vi "get_map_size.vi"(8 "error in (no error)":errorcluster, 10 "appended path":path, 11 "IntensityGraph in":refnum<vi>) -> (0 "error out":errorcluster, 2 "map size":cluster{dbl, dbl, dbl, dbl})   [LabVIEW 2012]
uses:
  <vilib>/Analysis/6fits.llb/Curve Fitting Criteria.ctl
  <vilib>/Utility/file.llb/Read From Spreadsheet File (string).vi
  <vilib>/Analysis/baseanly.llb/Mean (DBL).vi
  <vilib>/regexp/Match Regular Expression.xnode
  <vilib>/Analysis/NI_AALBase.lvlib
  <vilib>/Analysis/NI_AALPro.lvlib
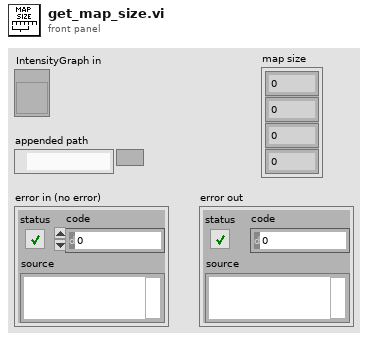
[diagram p1: front panel]
types:
  T1 = typedef "NI_AALPro.lvlib/Curve Fitting Criteria.ctl" = u16
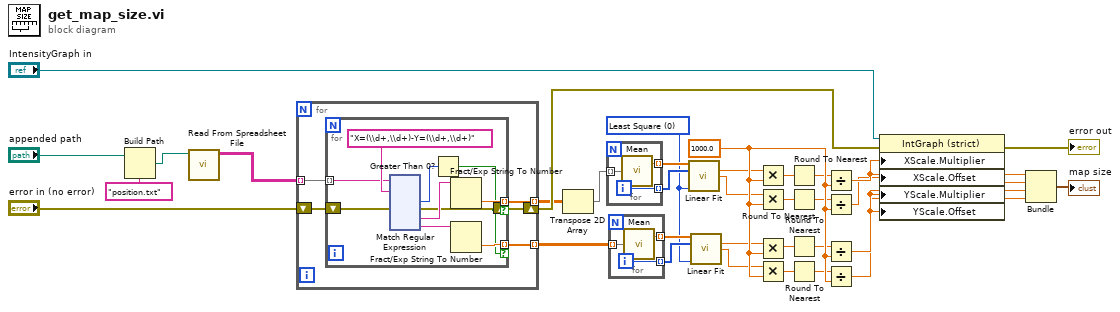
[diagram p0: block diagram]
diagram:
  w32 = 1000.0 ("y")
  w6 = T1 0 items=["Least Square", "Least Absolute Residual", "Bisquare"] ("method")
  n1 = Build Path(base path="appended path", name or relative path="position.txt") -> (appended path=w8:path)
  n2 = call-poly <vilib>:"Read From Spreadsheet File.vi"("file path (dialog if empty)"=w8) -> ("all rows"=w10:string[][])  [unwired: 6 in, 4 out]
  n3 = for {
    tunnel: w10 -> [w39] mode=indexing
    tunnel: [w38] -> w15 mode=indexing
    tunnel: [w37] -> w13 mode=indexing
    shift-right: [w36] -> w27
    shift-left: "error in (no error)" -> [w35]
    n4 = for {
      tunnel: w39 -> [w48] mode=indexing
      tunnel: [w46] -> w38 mode=indexing if=w42
      tunnel: [w45] -> w37 mode=indexing if=w42
      shift-right: [w41] -> w36
      shift-left: w35 -> [w40]
      n5 = xnode "Match Regular Expression"("input string"=w48, "regular expression"="X=(\\d+,\\d+)-Y=(\\d+,\\d+)", "error in"=w40) -> ("offset past match"=w43:i32, "error out"=w41:errorcluster, "submatch 1"=w44:string, "submatch 2"=w47:string)  [unwired: 3 in, 3 out]
      n6 = Greater Than 0?(x=w43) -> (x > 0?=w42:bool)
      n7 = Fract/Exp String To Number(string=w44) -> (number=w46:dbl)  [unwired: 3 in, 1 out]
      n8 = Fract/Exp String To Number(string=w47) -> (number=w45:dbl)  [unwired: 3 in, 1 out]
    }
  }
  n9 = Transpose 2D Array(2D array=w15) -> (transposed array=w14:dbl[][])
  n10 = for {
    tunnel: w14 -> [w166] mode=indexing
    tunnel: [w165] -> w17 mode=indexing
    tunnel: [w164] -> w11 mode=indexing
    i -> [w164]
    n11 = call-poly <vilib>:"Mean.vi"("X"=w166) -> ("mean"=w165:dbl)  [unwired: 1 out]
  }
  n12 = for {
    tunnel: w13 -> [w169] mode=indexing
    tunnel: [w168] -> w16 mode=indexing
    tunnel: [w167] -> w12 mode=indexing
    i -> [w167]
    n13 = call-poly <vilib>:"Mean.vi"("X"=w169) -> ("mean"=w168:dbl)  [unwired: 1 out]
  }
  n14 = call <vilib>:"Linear Fit.vi"("Y"=w17, "X"=w11, "method"=w6) -> ("slope"=w18:dbl, "intercept"=w19:dbl)  [unwired: 8 in, 3 out]
  n15 = call <vilib>:"Linear Fit.vi"("Y"=w16, "X"=w12, "method"=w6) -> ("slope"=w20:dbl, "intercept"=w21:dbl)  [unwired: 8 in, 3 out]
  n16 = Multiply(x=w18, y=w32) -> (x*y=w22:dbl)
  n17 = Multiply(x=w19, y=w32) -> (x*y=w23:dbl)
  n18 = Multiply(x=w20, y=w32) -> (x*y=w25:dbl)
  n19 = Multiply(x=w21, y=w32) -> (x*y=w24:dbl)
  n20 = Round To Nearest(number=w22) -> (nearest integer value=w28:dbl)
  n21 = Round To Nearest(number=w23) -> (nearest integer value=w29:dbl)
  n22 = Round To Nearest(number=w25) -> (nearest integer value=w30:dbl)
  n23 = Round To Nearest(number=w24) -> (nearest integer value=w31:dbl)
  n24 = Divide(x=w28, y=w32) -> (x/y=w5:dbl)
  n25 = Divide(x=w29, y=w32) -> (x/y=w4:dbl)
  n26 = Divide(x=w30, y=w32) -> (x/y=w3:dbl)
  n27 = Divide(x=w31, y=w32) -> (x/y=w2:dbl)
  n28 = property on="Property Node" class="IntGraph (strict)"(reference="IntensityGraph in", error in=w27, "XScale.Multiplier"=w5, "XScale.Offset"=w4, "YScale.Multiplier"=w3, "YScale.Offset"=w2) -> (error out=→"error out":errorcluster)  [unwired: 1 out]
  n29 = Bundle(w5, w4, w3, w2) -> (→"map size":cluster{dbl, dbl, dbl, dbl})  [unwired: 1 in]
